vi "Short_puff.vi"() -> (5 "Plug in titles":string[](array[string]), 7 "Plug in values":string[](array[string]))   [LabVIEW 2010]
uses:
  Controls/Post_Process.ctl
  Controls/Multi_run_mode.ctl
  Globals/Plug_in_data_global.vi
  Globals/Meas_global.vi
  Globals/Trav_pos_global.vi
  <vilib>/Analysis/NI_AALPro.lvlib
panel:
  out "Current Block No":i32
  in  "Save averaged traces?":bool
  in  "Save Block Time Trace?":bool
  in  "Pause Mode":T1(ring)
  in  "OK":bool
  out "Fall Traces":dbl
  out "Rise Traces":dbl
  out "Top 2":dbl(graph)
  out "Fall Time":dbl(graph)
  out "Delay 2":dbl(graph)
  out "Top":dbl(graph)
  out "Rise time":dbl(graph)
  out "Delay":dbl(graph)
  out "millisecond timer value":u32
  out "Fall Trace":cluster{dbl, dbl, dbl[]}(graph)
  out "Rise Trace":cluster{dbl, dbl, dbl[]}(graph)
  out "Source Off":i32
  out "Source On":i32
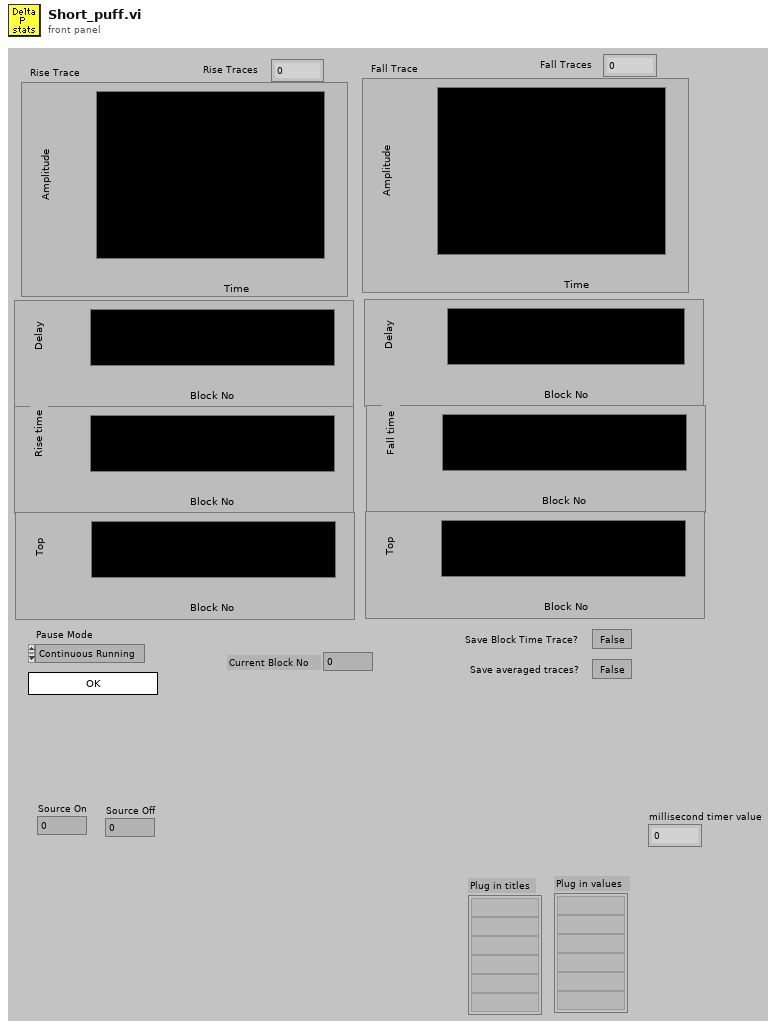
[diagram p1: front panel]
types:
  T1 = enum16{"Continuous Running", "After Each  Block"}
  T2 = typedef "Post_Process.ctl" = enum16{"Take New Data", "Post Process Raw Data File"}
  T3 = typedef "Multi_run_mode.ctl" = enum16{"Move Traverse Only", "Set Tunnel Speed Only", "Set Source Only", "Set Measurement Conditions", "Single Measurement", "Vertical Profile", "Lateral Profile", "Longitudinal Profile", "Explore Volume", "Multi-Axis Profile", "Auto Calibrate", "Meas Fast FID Bkgnd", "Check Beam Power", "Scanning Valve Measurement", "Run VI Named:", "Set ADAM Ch", "Wait (minutes)", "Send Message", "Synchronize With:", "Fall Back to this Row", "Turn Off Row Repeating", "Blank Row"}
  T4 = typedef "Traverse_cluster.ctl" = cluster{"Start X":dbl, "Start Y":dbl, "Start Z":dbl, "End X":dbl, "End Y":dbl, "End Z":dbl, "No. of pts.":i32, "Spacing":T5, "Filename":path, "Tunnel Speed":dbl, "Averaging time (min)":dbl, "Extra Commands":string, "Specific Arguments":string, "Emission Rate (l/min)":dbl, "Trace Gas Concentration (%)":dbl, "Density Ratio":string, "Comments":string, "Row No":i32, "Row Type Selector":T3, "Completion time":string, "Row Duration (mins)":dbl, "No. of Valid pts.":i32, "Meas Setup File":string}
  T5 = typedef "Spacing.ctl" = enum16{"Linear", "Log", "Gauss", "Specified", "N/A"}
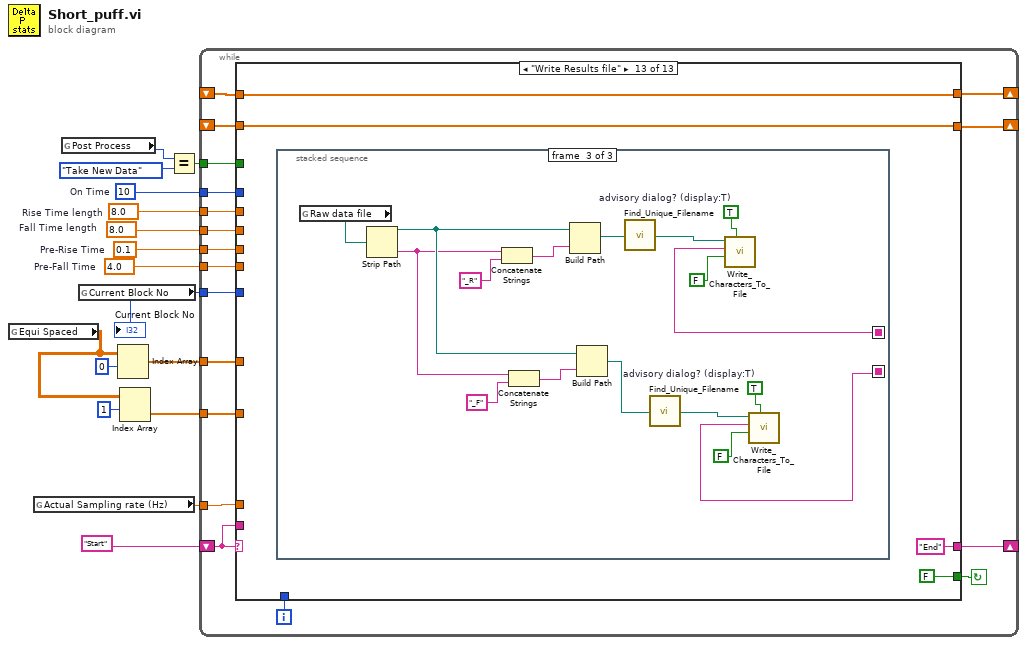
[diagram p0: block diagram]
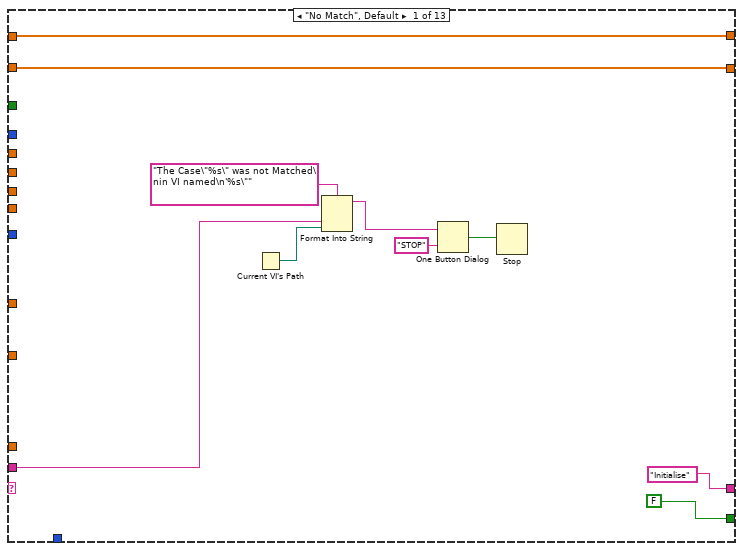
[diagram p2: hidden frame]
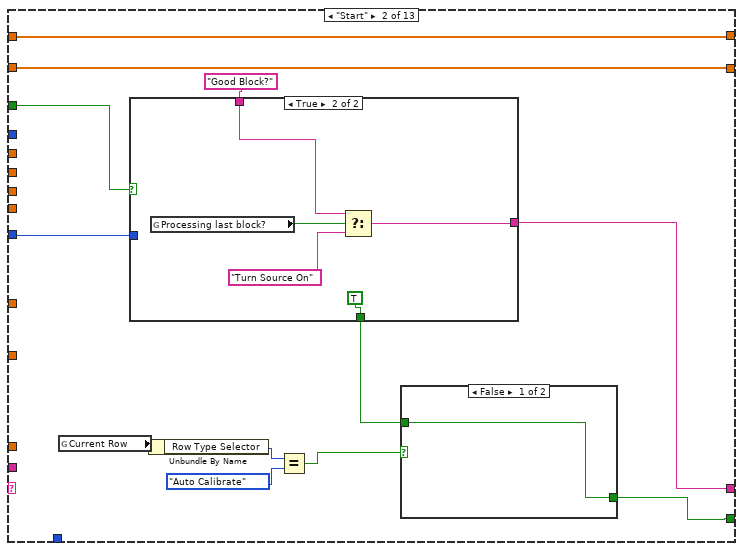
[diagram p3: hidden frame]
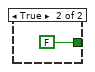
[diagram p4: hidden frame]
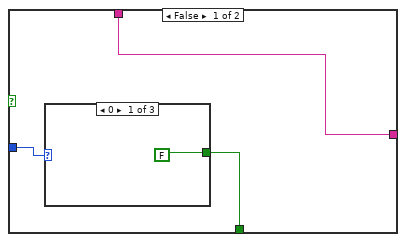
[diagram p5: hidden frame]
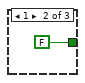
[diagram p6: hidden frame]
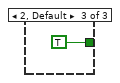
[diagram p7: hidden frame]
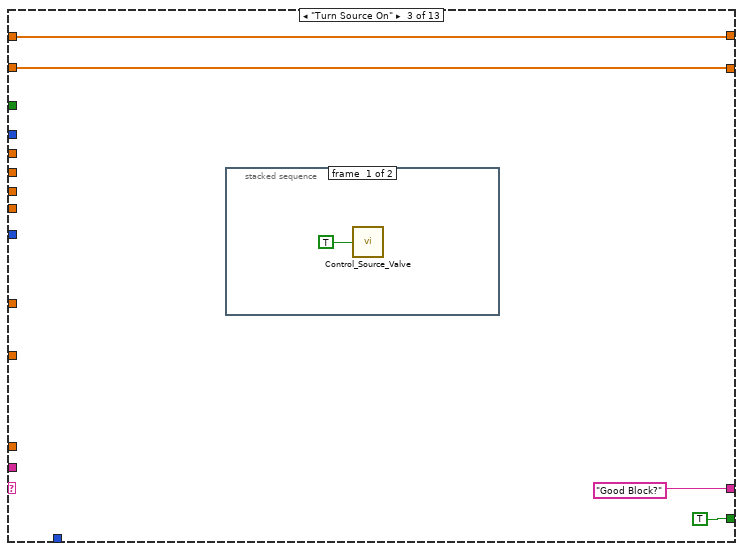
[diagram p8: hidden frame]
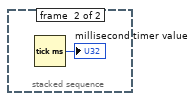
[diagram p9: hidden frame]
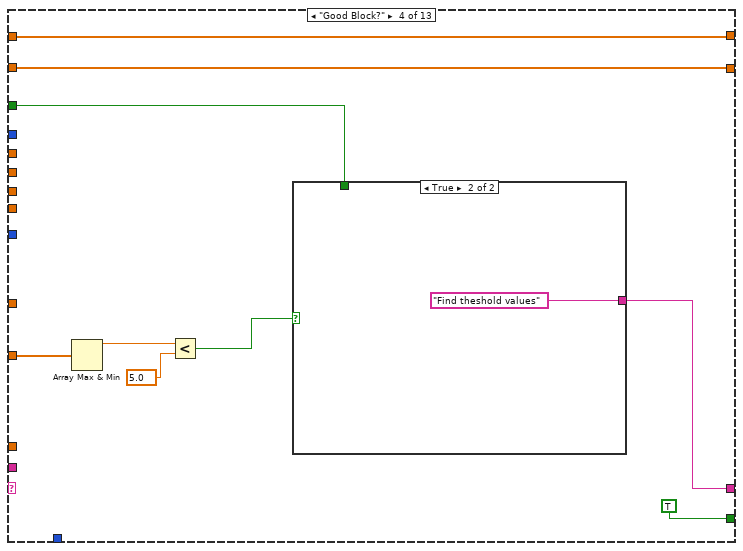
[diagram p10: hidden frame]
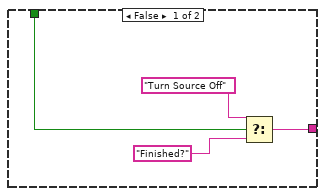
[diagram p11: hidden frame]
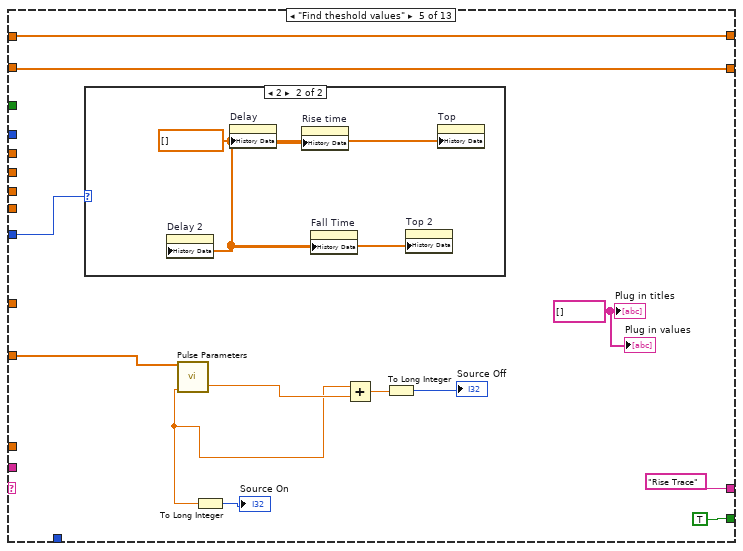
[diagram p12: hidden frame]
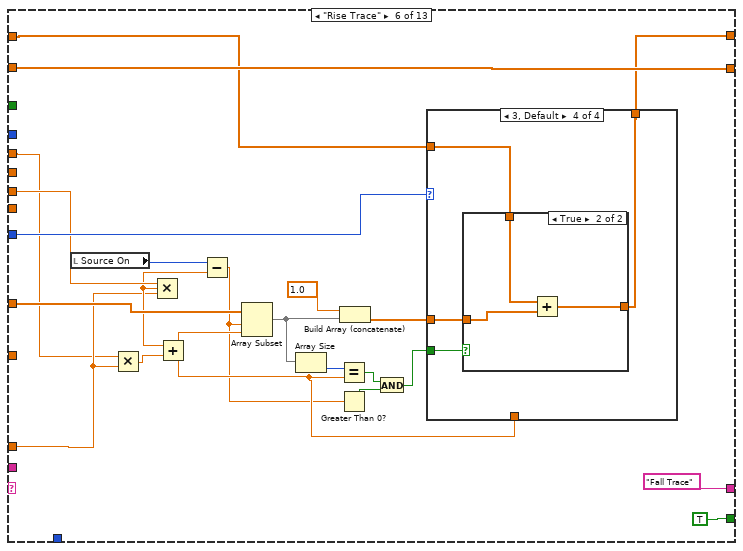
[diagram p14: hidden frame]
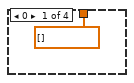
[diagram p15: hidden frame]
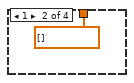
[diagram p16: hidden frame]
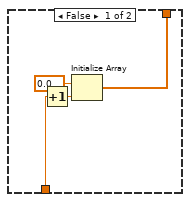
[diagram p18: hidden frame]
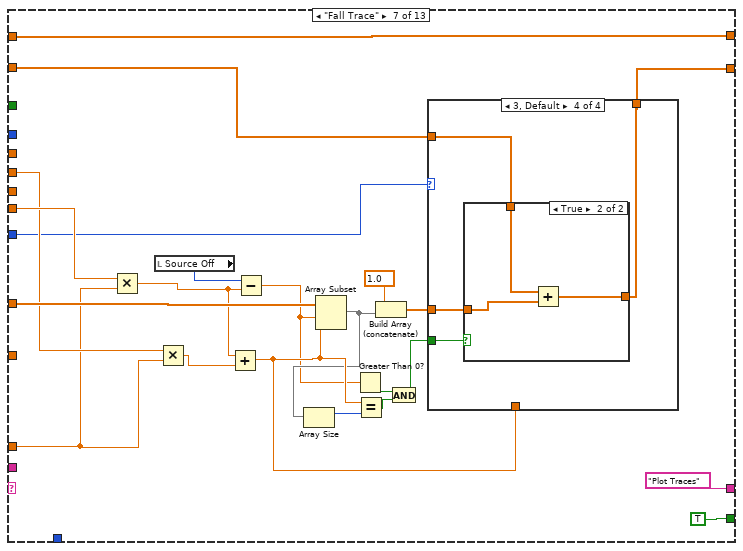
[diagram p20: hidden frame]
diagram:
  w1 = 0.1  # Pre-Rise Time
  w2 = 10  # On Time
  w7 = 4.0  # Pre-Fall Time
  w6 = 8.0  # Fall Time length
  w15 = 8.0  # Rise Time length
  n1 = global read "Plug_in_data_global.vi" "Equi Spaced"() -> (w14:dbl[][])
  n2 = global read "Meas_global.vi" "Actual Sampling rate (Hz)"() -> (w9:dbl)
  n3 = global read "Meas_global.vi" "Post Process"() -> (w4:T2)
  n4 = global read "Meas_global.vi" "Current Block No"() -> (w8:i32)
  "Current Block No" <- w8
  n5 = Index Array(array=w14, index (row)=0) -> (element=w10:dbl[])  [unwired: 1 in]
  n6 = Index Array(array=w14, index (row)=1) -> (element=w11:dbl[])  [unwired: 1 in]
  n7 = Equal?(x=w4, y=Post_Process."Take New Data" ("Post Process")) -> (x = y?=w3:bool)
  n8 = while {
    shift-left: "Start" -> [w32]
    shift-right: [w33] -> _
    shift-right: [w31] -> _
    shift-left: _ -> [w28]
    shift-right: [w30] -> _
    shift-left: _ -> [w29]
    tunnel: w15 -> [w27]
    tunnel: w11 -> [w26]
    tunnel: w10 -> [w25]
    tunnel: w9 -> [w24]
    tunnel: w8 -> [w23]
    tunnel: w7 -> [w22]
    tunnel: w6 -> [w21]
    tunnel: w3 -> [w20]
    tunnel: w2 -> [w19]
    tunnel: w1 -> [w18]
    i -> [w17]
    stop <- w34 continue-if-true
    n9 = case shown="\"Write Results file\"" w32 {
      tunnel: [FALSE w46 TRUE ("Processing last block?") TRUE TRUE ("Processing last block?") TRUE ("Processing last block?") TRUE ("Processing last block?") TRUE ("Processing last block?") FALSE ("Processing last block?") TRUE ("Processing last block?") TRUE ("Processing last block?") w292 FALSE ("Processing last block?")] -> w34
      tunnel: ["Initialise" w55 "Good Block?" w78 "Rise Trace" "Fall Trace" "Plot Traces" w197 "End" w242 "Save Rise and fall traces?" "Write Results file" "End"] -> w33
      tunnel: w32 -> [w39 _ _ _ _ _ _ _ _ _ _ _ _]
      tunnel: [w36 w54 w73 w84 w100 w120 w162 w208 w224 w246 w264 w297 w301] -> w31
      tunnel: [w35 w53 w72 w83 w95 w122 w153 w203 w223 w245 w263 w296 w300] -> w30
      tunnel: w29 -> [w35 w53 w72 w83 w95 w122 w154 w203 w223 w245 w263 w296 w300]
      tunnel: w28 -> [w36 w54 w73 w84 w100 w119 w162 w208 w224 w246 w264 w297 w301]
      tunnel: w27 -> [_ _ _ _ _ w107 _ _ _ _ _ _ _]
      tunnel: w26 -> [_ _ _ w82 w96 _ _ _ _ _ w260 _ _]
      tunnel: w25 -> [_ _ _ _ _ w121 w163 _ _ _ w259 _ _]
      tunnel: w24 -> [_ _ _ _ _ w108 w148 w193 _ _ _ _ _]
      tunnel: w23 -> [_ w51 _ _ w90 w118 w152 _ _ _ w258 _ _]
      tunnel: w22 -> [_ _ _ _ _ _ w160 w192 _ _ _ _ _]
      tunnel: w21 -> [_ _ _ _ _ _ w159 _ _ _ _ _ _]
      tunnel: w20 -> [_ w56 _ w77 _ _ _ w218 _ w238 _ _ _]
      tunnel: w19 -> [_ _ _ _ _ _ _ _ w220 _ _ _ _]
      tunnel: w18 -> [_ _ _ _ _ w113 _ w185 _ _ _ _ _]
      tunnel: w17 -> [_ _ _ _ _ _ _ _ _ w236 _ _ _]
      frame "No Match", Default {
        n10 = Current VI's Path() -> (path=w38:path)
        n11 = Format Into String(format string="The Case\"%s\" was not Matched\nin VI named\n'%s\"" ("Format String"), w39, w38) -> (resulting string=w42:string)  [unwired: 2 in, 1 out]
        n12 = One Button Dialog(message=w42, button name ("OK")="STOP") -> (true=w40:bool)
        n13 = Stop(stop? (T)=w40) -> ()
      }
      frame "Start" {
        n14 = global read "Trav_pos_global.vi" "Current Row"() -> (w50:T4)
        n15 = case shown="True" w56 {
          tunnel: [w61 w68] -> w55
          tunnel: "Good Block?" -> [w61 w67]
          tunnel: w51 -> [w60 _]
          tunnel: [w59 TRUE] -> w45
          frame False {
            n16 = case shown="0" w60 {
              tunnel: [FALSE FALSE TRUE] -> w59
              frame 0 {
              }
              frame 1 {
              }
              frame 2, Default {
              }
            }
          }
          frame True {
            n17 = global read "Meas_global.vi" "Processing last block?"() -> (w69:bool)
            n18 = Select(t=w67, s=w69, f="Turn Source On") -> (s? t:f=w68:string)
          }
        }
        n19 = Unbundle By Name(w50) -> ("Row Type Selector"=w48:T3)
        n20 = Equal?(x=w48, y=Multi_run_mode."Auto Calibrate" ("Row Type Selector")) -> (x = y?=w47:bool)
        n21 = case shown="False" w47 {
          tunnel: [w57 FALSE] -> w46
          tunnel: w45 -> [w57 _]
          frame False {
          }
          frame True {
          }
        }
      }
      frame "Turn Source On" {
        n22 = stacked-sequence {
          frame #0 {
            n23 = call "Control_Source_Valve.vi"("Source Valve"=TRUE) -> ()  [unwired: 2 out]
          }
          frame #1 {
            n24 = Tick Count (ms)() -> (millisecond timer value=→"millisecond timer value":u32)
          }
        }
      }
      frame "Good Block?" {
        n25 = Array Max & Min(array=w82) -> (max value=w81:dbl)  [unwired: 3 out]
        n26 = Less?(x=w81, y=5.0) -> (x < y?=w79:bool)
        n27 = case shown="True" w79 {
          tunnel: [w86 "Find theshold values"] -> w78
          tunnel: w77 -> [w88 _]
          frame False {
            n28 = Select(t="Turn Source Off", s=w88, f="Finished?") -> (s? t:f=w86:string)
          }
          frame True {
          }
        }
      }
      frame "Find theshold values" {
        w91 = string[] [] ("Plug in titles")
        n29 = case shown="2" w90 {
          frame 0, Default {
          }
          frame 2 {
            w102 = dbl[] [] ("History Data")
            n30 = property on="Delay 2" class="WFChart (strict)"("History Data"=w102) -> ()  [unwired: 2 in, 2 out]
            n31 = property on="Delay" class="WFChart (strict)"("History Data"=w102) -> ()  [unwired: 2 in, 2 out]
            n32 = property on="Rise time" class="WFChart (strict)"("History Data"=w102) -> ()  [unwired: 2 in, 2 out]
            n33 = property on="Fall Time" class="WFChart (strict)"("History Data"=w102) -> ()  [unwired: 2 in, 2 out]
            n34 = property on="Top 2" class="WFChart (strict)"("History Data"=w102) -> ()  [unwired: 2 in, 2 out]
            n35 = property on="Top" class="WFChart (strict)"("History Data"=w102) -> ()  [unwired: 2 in, 2 out]
          }
        }
        n36 = call <vilib>:"Pulse Parameters.vi"("X"=w96) -> ("delay"=w98:dbl, "duration"=w99:dbl)  [unwired: 4 in, 9 out]
        n37 = To Long Integer(number=w98) -> (32bit integer=→"Source On":i32)
        n38 = Add(x=w98, y=w99) -> (x+y=w97:dbl)
        n39 = To Long Integer(number=w97) -> (32bit integer=→"Source Off":i32)
        "Plug in values" <- w91
        "Plug in titles" <- w91
      }
      frame "Rise Trace" {
        n40 = local read "Source On"() -> (w112:i32)
        n41 = Multiply(x=w107, y=w108) -> (x*y=w111:dbl)
        n42 = Multiply(x=w113, y=w108) -> (x*y=w110:dbl)
        n43 = Add(x=w110, y=w111) -> (x+y=w109:dbl)
        n44 = Subtract(x=w112, y=w110) -> (x-y=w106:dbl)
        n45 = Array Subset(array=w121, index=w106, length=w109) -> (w116:dbl[])
        n46 = Array Size(array=w116) -> (size(s)=w117:i32)
        n47 = Equal?(x=w117, y=w109) -> (x = y?=w105:bool)
        n48 = Greater Than 0?(x=w106) -> (x > 0?=w104:bool)
        n49 = Build Array (concatenate)(1.0, w116) -> (w114:dbl[])
        n50 = And(x=w105, y=w104) -> (x .and. y?=w103:bool)
        n51 = case shown="3, Default" w118 {
          tunnel: [dbl[] [] dbl[] [] w128 w137] -> w120
          tunnel: w114 -> [_ _ w127 w139]
          tunnel: w119 -> [_ _ _ w138]
          tunnel: w103 -> [_ _ w130 w136]
          tunnel: w109 -> [_ _ w129 _]
          frame 0 {
          }
          frame 1 {
          }
          frame 2 {
            n52 = case shown="True" w130 {
              tunnel: w129 -> [w134 _]
              tunnel: [w132 w135] -> w128
              tunnel: w127 -> [_ w135]
              frame False {
                n53 = Increment(x=w134) -> (x+1=w131:dbl)
                n54 = Initialize Array(0.0 ("element"), w131) -> (w132:dbl[])
              }
              frame True {
              }
            }
          }
          frame 3, Default {
            n55 = case shown="True" w136 {
              tunnel: w139 -> [_ w143]
              tunnel: w138 -> [w140 w142]
              tunnel: [w140 w141] -> w137
              frame False {
              }
              frame True {
                n56 = Add(x=w142, y=w143) -> (x+y=w141:dbl[])
              }
            }
          }
        }
      }
      frame "Fall Trace" {
        n57 = Multiply(x=w160, y=w148) -> (x*y=w158:dbl)
        n58 = local read "Source Off"() -> (w161:i32)
        n59 = Multiply(x=w159, y=w148) -> (x*y=w157:dbl)
        n60 = Add(x=w158, y=w157) -> (x+y=w155:dbl)
        n61 = Subtract(x=w161, y=w158) -> (x-y=w147:dbl)
        n62 = Array Subset(array=w163, index=w147, length=w155) -> (w150:dbl[])
        n63 = Array Size(array=w150) -> (size(s)=w156:i32)
        n64 = Greater Than 0?(x=w147) -> (x > 0?=w145:bool)
        n65 = Equal?(x=w155, y=w156) -> (x = y?=w146:bool)
        n66 = Build Array (concatenate)(1.0, w150) -> (w149:dbl[])
        n67 = And(x=w145, y=w146) -> (x .and. y?=w144:bool)
        n68 = case shown="3, Default" w152 {
          tunnel: [dbl[] [] dbl[] [] w169 w178] -> w153
          tunnel: w149 -> [_ _ w168 w180]
          tunnel: w154 -> [_ _ _ w179]
          tunnel: w144 -> [_ _ w171 w177]
          tunnel: w155 -> [_ _ w170 _]
          frame 0 {
          }
          frame 1 {
          }
          frame 2 {
            n69 = case shown="False" w171 {
              tunnel: w170 -> [w175 _]
              tunnel: [w173 w176] -> w169
              tunnel: w168 -> [_ w176]
              frame False {
                n70 = Increment(x=w175) -> (x+1=w172:dbl)
                n71 = Initialize Array(0.0 ("element"), w172) -> (w173:dbl[])
              }
              frame True {
              }
            }
          }
          frame 3, Default {
            n72 = case shown="True" w177 {
              tunnel: w180 -> [_ w184]
              tunnel: w179 -> [w181 w183]
              tunnel: [w181 w182] -> w178
              frame False {
              }
              frame True {
                n73 = Add(x=w183, y=w184) -> (x+y=w182:dbl[])
              }
            }
          }
        }
      }
      frame "Plot Traces" {
        n74 = Reciprocal(x=w193) -> (1/x=w191:dbl)
        n75 = global read "Meas_global.vi" "Processing last block?"() -> (w219:bool)
        n76 = Array Subset(array=w208, index=1) -> (w207:dbl[])  [unwired: 1 in]
        n77 = Index Array(array=w208, index=0) -> (element=w206:dbl)
        "Rise Traces" <- w206
        n78 = Array Subset(array=w203, index=1) -> (w202:dbl[])  [unwired: 1 in]
        n79 = Index Array(array=w203, index=0) -> (element=w201:dbl)
        "Fall Traces" <- w201
        n80 = Negate(x=w185) -> (-x=w187:dbl)
        n81 = To Double Precision Float(number=w192) -> (double precision float=w188:dbl)
        n82 = Divide(x=w202, y=w201) -> (x/y=w190:dbl[])
        n83 = Reverse 1D Array(array=w190) -> (reversed array=w213:dbl[])
        n84 = Divide(x=w207, y=w206) -> (x/y=w195:dbl[])
        n85 = Negate(x=w188) -> (-x=w186:dbl)
        n86 = Compound Arithmetic op=AND(invert w219, w218) -> (w199:bool)
        n87 = Bundle(w187, w191, w195) -> (→"Rise Trace":cluster{dbl, dbl, dbl[]})  [unwired: 1 in]
        n88 = Bundle(w186, w191, w190) -> (→"Fall Trace":cluster{dbl, dbl, dbl[]})  [unwired: 1 in]
        n89 = call <vilib>:"Pulse Parameters.vi"("X"=w195) -> ("risetime"=→"Rise time":dbl, "top"=→"Top":dbl, "delay"=→"Delay":dbl)  [unwired: 4 in, 8 out]
        n90 = call <vilib>:"Pulse Parameters.vi"("X"=w213) -> ("risetime"=→"Fall Time":dbl, "top"=→"Top 2":dbl, "delay"=→"Delay 2":dbl)  [unwired: 4 in, 8 out]
        n91 = Select(t="Turn Source Off", s=w199, f="Finished?") -> (s? t:f=w197:string)
      }
      frame "Turn Source Off" {
        n92 = stacked-sequence {
          tunnel: w220 -> [w229 _]
          frame #0 {
            n93 = local read "millisecond timer value"() -> (w230:u32)
            n94 = Tick Count (ms)() -> (millisecond timer value=w231:u32)
            n95 = Subtract(x=w231, y=w230) -> (x-y=w226:u32)
            n96 = Multiply(x=1000, y=w229) -> (x*y=w227:i32)
            n97 = Subtract(x=w227, y=w226) -> (x-y=w225:u32)
            n98 = Wait (ms)(milliseconds to wait=w225) -> ()  [unwired: 1 out]
          }
          frame #1 {
            n99 = call "Control_Source_Valve.vi"("Source Valve"=FALSE) -> ()  [unwired: 2 out]
          }
        }
      }
      frame "Finished?" {
        n100 = Quotient & Remainder(x=w236, y=50) -> (x-y*floor(x/y)=w234:i32)  [unwired: 1 out]
        n101 = Equal To 0?(x=w234) -> (x = 0?=w233:bool)
        n102 = case shown="False" w233 {
          frame False {
          }
          frame True {
            n103 = Current VI's Path() -> (path=w247:path)
            n104 = call "Bring_to_front.vi"("path"=w247) -> ()
          }
        }
        n105 = case shown="\"Continuous Running\"" "Pause Mode" {
          tunnel: [TRUE "OK"] -> w239
          tunnel: [FALSE TRUE] -> w240
          frame "Continuous Running" {
          }
          frame "After Each  Block" {
            n106 = Wait (ms)(milliseconds to wait=u32 100 ("f")) -> ()  [unwired: 1 out]
          }
        }
        n107 = Or(x=w239, y=w238) -> (x .or. y?=w237:bool)
        n108 = property on="OK" class="Bool"("Visible"=w240) -> ()  [unwired: 2 in, 2 out]
        n109 = case shown="True" w237 {
          tunnel: "Save Block Time Trace?" -> [_ w257]
          tunnel: ["Finished?" w255] -> w242
          frame False {
          }
          frame True {
            n110 = Select(t="Save Block time trace", s=w257, f="Save Rise and fall traces?") -> (s? t:f=w255:string)
          }
        }
      }
      frame "Save Block time trace" {
        n111 = stacked-sequence {
          seq-local: [w268 _] -> [_ w286]
          tunnel: w260 -> [w267 _]
          tunnel: w259 -> [w266 _]
          tunnel: w258 -> [_ w283]
          frame #0 {
            n112 = for {
              tunnel: w267 -> [w278] mode=indexing
              tunnel: w266 -> [w277] mode=indexing
              tunnel: [w276] -> w265 mode=indexing
              n113 = Number To Fractional String(number=w277, precision (6)=i16 3) -> (F-format string=w275:string)  [unwired: 2 in]
              n114 = Number To Fractional String(number=w278, precision (6)=i16 1) -> (F-format string=w274:string)  [unwired: 2 in]
              n115 = Build Array(w274, w275) -> (w276:string[])
            }
            n116 = Build Array("Source:Valve:Voltage", "FFID:Concentration:C (ppm)") -> (w271:string[])
            n117 = Build Array (concatenate)(w271, w265) -> (w270:string[][])
            n118 = Array To Spreadsheet String(array=w270, 3:"%s" ("format string")) -> (spreadsheet string=w268:string)  [unwired: 1 in]
          }
          frame #1 {
            w288 = TRUE  # advisory dialog? (display:T)
            n119 = global read "Meas_global.vi" "Raw data file"() -> (w291:path)
            n120 = Strip Path(path=w291) -> (stripped path=w285:path, name=w284:string)
            n121 = Format Into String(format string="_B%d", initial string=w284, w283) -> (resulting string=w281:string)  [unwired: 1 in, 1 out]
            n122 = Build Path(base path=w285, name or relative path=w281) -> (appended path=w290:path)
            n123 = call "Find_Unique_Filename.vi"("Path In"=w290) -> ("Unique Path Out"=w289:path)  [unwired: 2 in]
            n124 = call "Write_Characters_To_File.vi"("file path (dialog if empty)"=w289, "advisory dialog? (display:T)"=w288, "character string"=w286, "append to file? (new file:F)"=FALSE) -> ()  [unwired: 4 in, 1 out]
          }
        }
      }
      frame "Save Rise and fall traces?" {
        n125 = global read "Meas_global.vi" "Processing last block?"() -> (w294:bool)
        n126 = And(x="Save averaged traces?", y=w294) -> (x .and. y?=w292:bool)
      }
      frame "Write Results file" {
        n127 = stacked-sequence {
          seq-local: [w302 _ _] -> [_ _ w346]
          seq-local: [_ w322 _] -> [_ _ w347]
          frame #0 {
            n128 = local read "Rise Trace"() -> (w314:cluster{dbl, dbl, dbl[]})
            n129 = Unbundle(w314) -> (w312:dbl, w313:dbl, w311:dbl[])
            n130 = for {
              tunnel: w313 -> [w320]
              tunnel: w312 -> [w319]
              tunnel: w311 -> [w315] mode=indexing
              tunnel: [w317] -> w309 mode=indexing
              i -> [w321]
              n131 = Multiply(x=w320, y=w321) -> (x*y=w318:dbl)
              n132 = Add(x=w319, y=w318) -> (x+y=w316:dbl)
              n133 = Build Array(w316, w315) -> (w317:dbl[])
            }
            n134 = Number To Fractional String(number=w309, precision (6)=i16 3) -> (F-format string=w308:string[][])  [unwired: 2 in]
            n135 = Build Array("Time:(s):T=0 when valve opened", "FFID:Concentration:C") -> (w305:string[])
            n136 = Build Array (concatenate)(w305, w308) -> (w304:string[][])
            n137 = Array To Spreadsheet String(array=w304, 3:"%s" ("format string")) -> (spreadsheet string=w302:string)  [unwired: 1 in]
          }
          frame #1 {
            n138 = local read "Fall Trace"() -> (w334:cluster{dbl, dbl, dbl[]})
            n139 = Unbundle(w334) -> (w332:dbl, w333:dbl, w331:dbl[])
            n140 = for {
              tunnel: w333 -> [w340]
              tunnel: w332 -> [w339]
              tunnel: w331 -> [w335] mode=indexing
              tunnel: [w337] -> w329 mode=indexing
              i -> [w341]
              n141 = Multiply(x=w340, y=w341) -> (x*y=w338:dbl)
              n142 = Add(x=w339, y=w338) -> (x+y=w336:dbl)
              n143 = Build Array(w336, w335) -> (w337:dbl[])
            }
            n144 = Number To Fractional String(number=w329, precision (6)=i16 3) -> (F-format string=w328:string[][])  [unwired: 2 in]
            n145 = Build Array("Time:(s):T=0 when valve opened", "FFID:Concentration:C") -> (w325:string[])
            n146 = Build Array (concatenate)(w325, w328) -> (w324:string[][])
            n147 = Array To Spreadsheet String(array=w324, 3:"%s" ("format string")) -> (spreadsheet string=w322:string)  [unwired: 1 in]
          }
          frame #2 {
            w348 = TRUE  # advisory dialog? (display:T)
            w351 = TRUE  # advisory dialog? (display:T)
            n148 = global read "Meas_global.vi" "Raw data file"() -> (w358:path)
            n149 = Strip Path(path=w358) -> (stripped path=w353:path, name=w352:string)
            n150 = Concatenate Strings(w352, "_R" ("string")) -> (w357:string)
            n151 = Concatenate Strings(w352, "_F" ("string")) -> (w354:string)
            n152 = Build Path(base path=w353, name or relative path=w357) -> (appended path=w343:path)
            n153 = Build Path(base path=w353, name or relative path=w354) -> (appended path=w345:path)
            n154 = call "Find_Unique_Filename.vi"("Path In"=w343) -> ("Unique Path Out"=w342:path)  [unwired: 2 in]
            n155 = call "Find_Unique_Filename.vi"("Path In"=w345) -> ("Unique Path Out"=w344:path)  [unwired: 2 in]
            n156 = call "Write_Characters_To_File.vi"("file path (dialog if empty)"=w342, "advisory dialog? (display:T)"=w351, "character string"=w346, "append to file? (new file:F)"=FALSE) -> ()  [unwired: 4 in, 1 out]
            n157 = call "Write_Characters_To_File.vi"("file path (dialog if empty)"=w344, "advisory dialog? (display:T)"=w348, "character string"=w347, "append to file? (new file:F)"=FALSE) -> ()  [unwired: 4 in, 1 out]
          }
        }
      }
    }
  }
